vi "Read Radius.vi"(8 "error in (no error)":errorcluster, 11 "CircleShape in":refnum<class "CircleShape.lvclass">) -> (0 "error out":errorcluster, 2 "Radius":i16, 3 "CircleShape out":refnum<class "CircleShape.lvclass">)   [LabVIEW 2022 SP3, in "CircleShape.lvclass"]
uses:
  CircleShape.lvclass
  CircleShape.lvclass/CircleShape.ctl
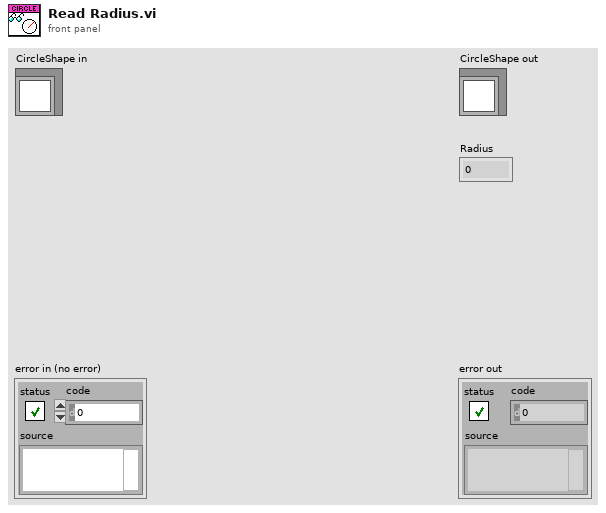
[diagram p1: front panel]
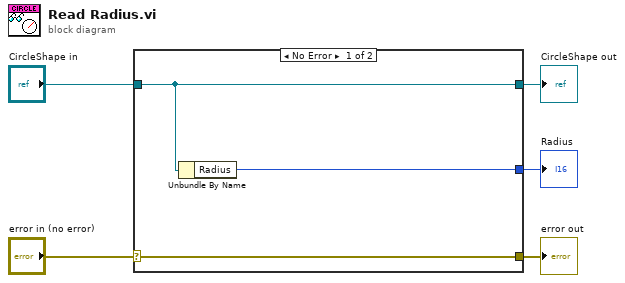
[diagram p0: block diagram]
diagram:
  n1 = case shown="No Error" "error in (no error)" {
    selector: "error in (no error)" -> [w8 w9]
    tunnel: [w8 w9] -> w4
    tunnel: [w7 w10] -> w2
    tunnel: "CircleShape in" -> [w7 w10]
    tunnel: [w6 _] -> w1
    frame No Error {
      n2 = Unbundle By Name(w7) -> ("Radius"=w6:i16)
    }
    frame Error {
    }
  }
  "error out" <- w4
  "CircleShape out" <- w2
  "Radius" <- w1
